vi "Match Block Upload Response.vi"(8 "error in":errorcluster, 10 "Frame Data":u8[](array[numeric]), 11 "Block Upload Initiate in":refnum<class "Block Upload Initiate Transfer.lvclass">) -> (0 "error out":errorcluster, 2 "Match":bool, 3 "SDO Transfer out":refnum<class "SDO Transfer.lvclass">)   [LabVIEW 2020, in "CANopen.lvlib" / "SDO Manager.lvlib" / "Block Upload Initiate Transfer.lvclass"]
uses:
  Block Upload Initiate Transfer.lvclass
  SDO Transfer/SDO Transfer.lvclass
  Block Upload Sub-Block Transfer/Block Upload Sub-Block Transfer.lvclass
  Block Upload Initiate Transfer.lvclass/Block Upload Initiate Transfer.ctl
  HAL/Source/Interfaces/ICommunicate/ICommunicate.lvclass
  D:/git/CANopen-LabVIEW/source/SDO/SDO Manager/SDO Transfer/SDO Transfer.lvclass
  D:/git/CANopen-LabVIEW/source/SDO/SDO Manager/Block Upload Initiate Transfer/Block Upload Initiate Transfer.lvclass
  D:/git/CANopen-LabVIEW/source/SDO/SDO Manager/Block Upload Sub-Block Transfer/Block Upload Sub-Block Transfer.lvclass
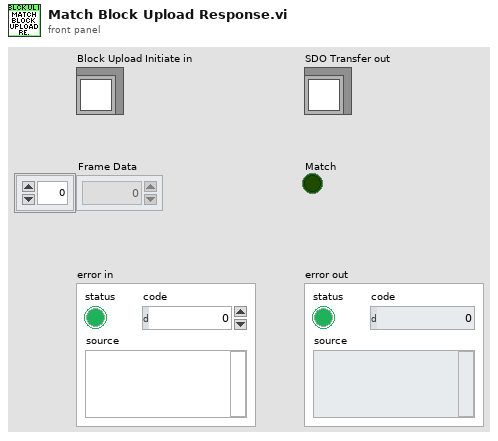
[diagram p1: front panel]
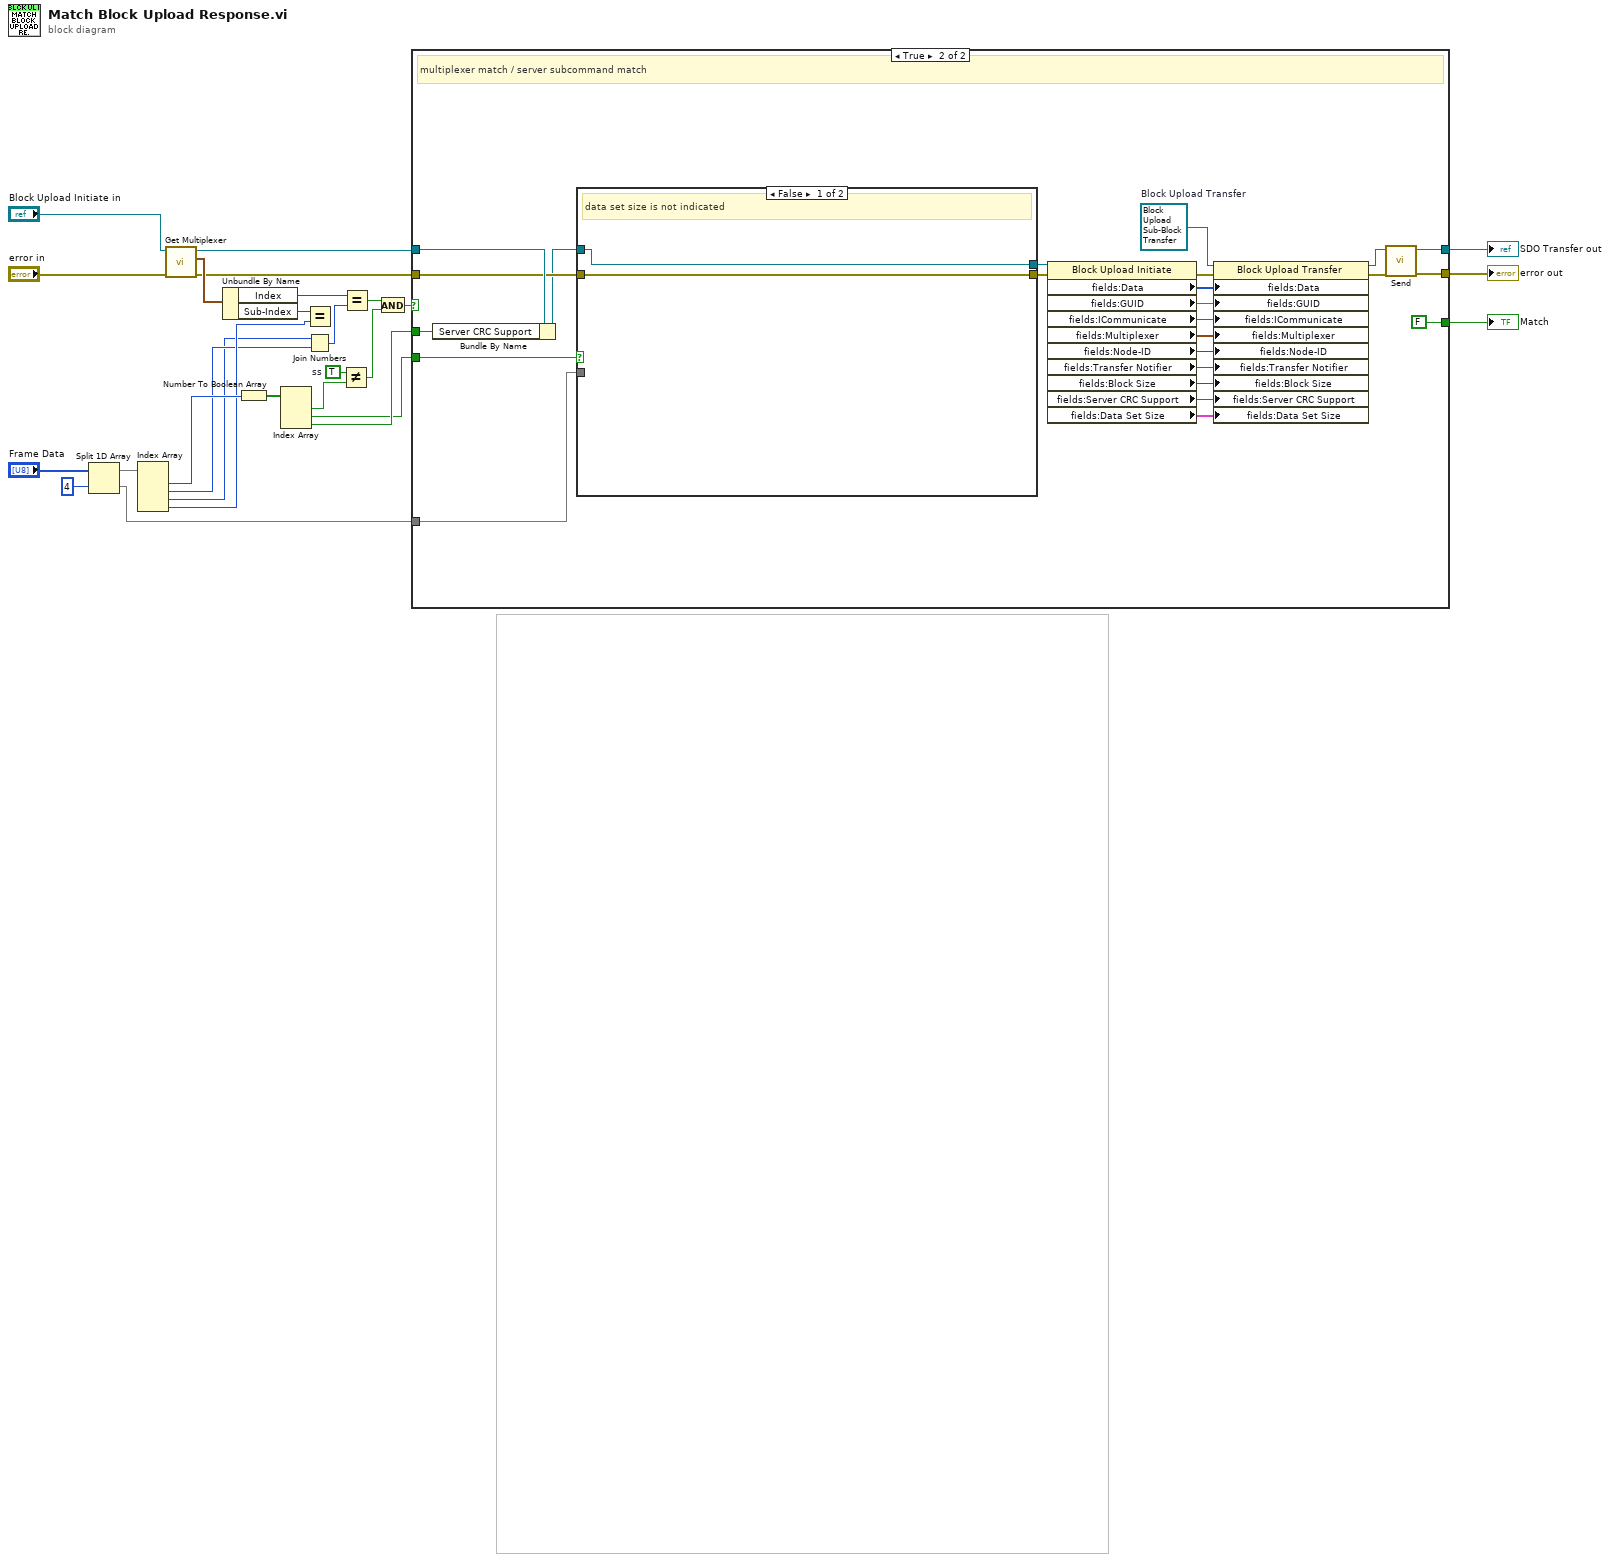
[diagram p0: block diagram]
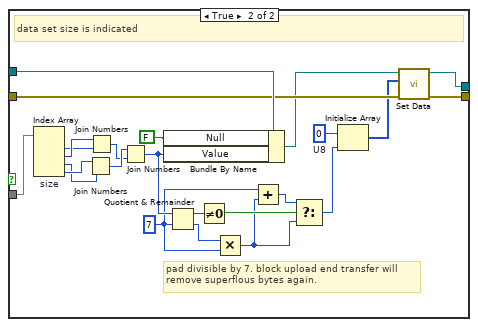
[diagram p3: hidden frame]
diagram:
  w20 = TRUE  # ss
  n1 = Split 1D Array(array="Frame Data", index=4) -> (first subarray=w7:u8[], second subarray=w4:u8[])
  n2 = Index Array(array=w7) -> (element #1=w6:u8, element #2=w2:u8, element #3=w1:u8, element #4=w3:u8)  [unwired: 4 in]
  n3 = call "Get Multiplexer.vi"("error in"="error in", "SDO Transfer in"="Block Upload Initiate in") -> ("error out"=w24:errorcluster, "Multiplexer"=w27:cluster{"Index":u16, "Sub-Index":u8}, "SDO Transfer out"=w26:refnum<class "Block Upload Initiate Transfer.lvclass">)  [unwired: 7 in]
  n4 = Unbundle By Name(w27) -> ("Index"=w13:u16, "Sub-Index"=w14:u8)
  n5 = Number To Boolean Array(number=w6) -> (Boolean array=w18:bool[])
  n6 = Index Array(array=w18) -> (element #1=w23:bool, element #2=w21:bool, element #3=w22:bool)  [unwired: 3 in]
  n7 = Equal?(x=w14, y=w3) -> ()  [unwired: 1 out]
  n8 = Join Numbers(hi=w1, lo=w2) -> ((hi.lo)=w15:u16)
  n9 = Not Equal?(x=w20, y=w23) -> (x != y?=w19:bool)
  n10 = Equal?(x=w13, y=w15) -> (x = y?=w16:bool)
  n11 = And(x=w16, y=w19) -> (x .and. y?=w17:bool)
  n12 = case shown="True" w17 {
    tunnel: w24 -> [w29 w51]
    tunnel: w26 -> [w28 w52]
    tunnel: [w28 w33] -> w10
    tunnel: [w29 w34] -> w11
    tunnel: [_ FALSE] -> w12
    tunnel: w4 -> [_ w53]
    tunnel: w21 -> [_ w49]
    tunnel: w22 -> [_ w48]
    frame False {
      # "no match"
    }
    frame True {
      w46 = refnum<class "Block Upload Sub-Block Transfer.lvclass"> refnum  # Block Upload Transfer
      # "multiplexer match / server subcommand match"
      n13 = Bundle By Name(cluster=w52, "Server CRC Support"=w48) -> (w50:refnum<class "Block Upload Initiate Transfer.lvclass">)
      n14 = case shown="False" w49 {
        tunnel: w53 -> [_ w76]
        tunnel: w50 -> [w54 w71]
        tunnel: w51 -> [w55 w69]
        tunnel: [w54 w66] -> w44
        tunnel: [w55 w68] -> w45
        frame False {
          # "data set size is not indicated"
        }
        frame True {
          w56 = u32 7 ("y")
          w64 = u8 0  # U8
          # "pad divisible by 7. block upload end transfer will\nremove superflous bytes again."
          # "data set size is indicated"
          n15 = Index Array "size"(array=w76) -> (element #1=w72:u8, element #2=w73:u8, element #3=w74:u8, element #4=w75:u8)  [unwired: 4 in]
          n16 = Join Numbers(hi=w75, lo=w74) -> ((hi.lo)=w78:u16)
          n17 = Join Numbers(hi=w73, lo=w72) -> ((hi.lo)=w77:u16)
          n18 = Join Numbers(hi=w78, lo=w77) -> ((hi.lo)=w63:u32)
          n19 = Bundle By Name(cluster=w71, "Null"=FALSE ("Data Set Size.Null"), "Value"=w63) -> (w67:refnum<class "Block Upload Initiate Transfer.lvclass">)
          n20 = Quotient & Remainder(x=w63, y=w56) -> (x-y*floor(x/y)=w62:u32, floor(x/y)=w59:u32)
          n21 = Not Equal To 0?(x=w62) -> (x != 0?=w61:bool)
          n22 = Multiply(x=w59, y=w56) -> (x*y=w57:u32)
          n23 = Add(x=w56, y=w57) -> (x+y=w58:u32)
          n24 = Select(t=w58, s=w61, f=w57) -> (s? t:f=w60:u32)
          n25 = Initialize Array(w64, w60) -> (w65:u8[])
          n26 = call "Set Data.vi"("error in"=w69, "Data"=w65, "SDO Transfer in"=w67) -> ("error out"=w68:errorcluster, "SDO Transfer out"=w66:refnum<class "Block Upload Initiate Transfer.lvclass">)  [unwired: 7 in]
        }
      }
      n27 = property class="Block Upload Initiate"(reference=w44, error in=w45) -> (error out=w43:errorcluster, "fields:Data"=w37:u8[], "fields:GUID"=w38:string, "fields:ICommunicate"=w39:refnum<class "ICommunicate.lvclass">, "fields:Multiplexer"=w40:cluster{"Index":u16, "Sub-Index":u8}, "fields:Node-ID"=w41:u8, "fields:Transfer Notifier"=w42:refnum<notifier>, "fields:Block Size"=w32:u8, "fields:Server CRC Support"=w31:bool, "fields:Data Set Size"=w30:cluster{"Null":bool, "Value":u32})  [unwired: 1 out]
      n28 = property class="Block Upload Transfer"(reference=w46, error in=w43, "fields:Data"=w37, "fields:GUID"=w38, "fields:ICommunicate"=w39, "fields:Multiplexer"=w40, "fields:Node-ID"=w41, "fields:Transfer Notifier"=w42, "fields:Block Size"=w32, "fields:Server CRC Support"=w31, "fields:Data Set Size"=w30) -> (reference out=w36:refnum<class "Block Upload Sub-Block Transfer.lvclass">, error out=w35:errorcluster)
      n29 = call-dynamic "Send.vi"("error in"=w35, "Block Upload Transfer in"=w36) -> ("error out"=w34:errorcluster, "Block Upload Transfer out"=w33:refnum<class "Block Upload Sub-Block Transfer.lvclass">)  [unwired: 8 in]
    }
  }
  "Match" <- w12
  "error out" <- w11
  "SDO Transfer out" <- w10
